vi "Test List Tests from lvlib.vi"(8 "error in (no error)":errorcluster, 11 "Test Case In":refnum<class "LUnit Test Suite Tests.lvclass">) -> (0 "error out":errorcluster, 3 "Test Case Out":refnum<class "LUnit Test Suite Tests.lvclass">)   [LabVIEW 2020, in "LUnit Test Suite Tests.lvclass"]
uses:
  LUnit Test Suite Tests.lvclass
  LUnit Test Suite Tests.lvclass/LUnit Test Suite Tests.ctl
  b74e4934-f044-4222-b3dd-fc90e6c1bd4f.vi
  source/API/Test Suite Factory/Test Suite Factory.lvclass
  source/API/LUnit Test Suite/LUnit Test Suite.lvclass
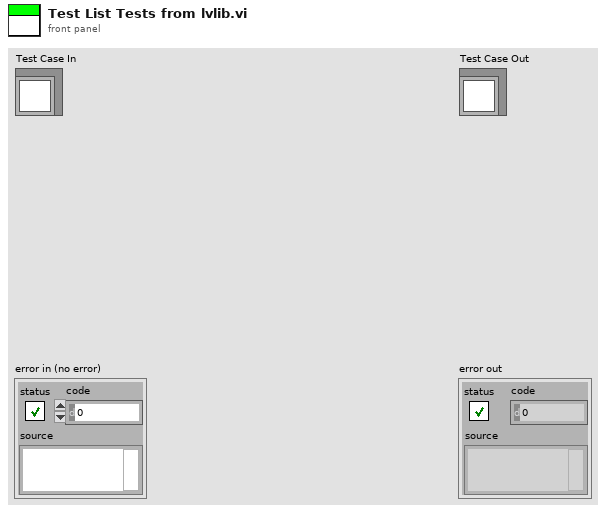
[diagram p1: front panel]
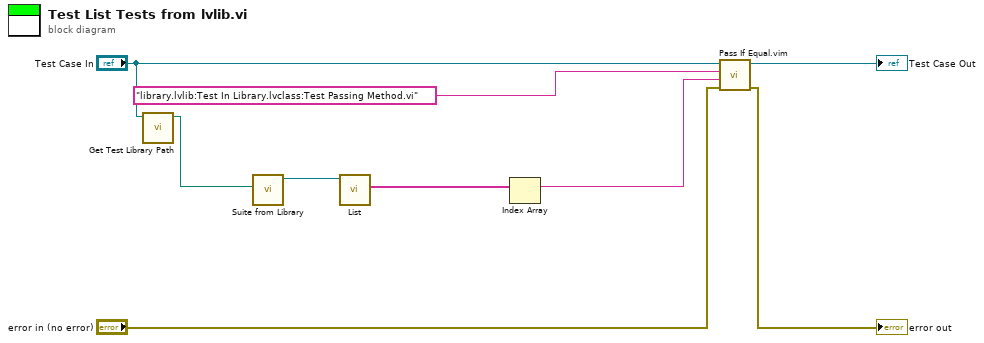
[diagram p0: block diagram]
diagram:
  n1 = call "Get Test Library Path.vi"("LUnit Test Suite Tests in"="Test Case In") -> ("lvlib path"=w1:path)  [unwired: 9 in, 1 out]
  n2 = call "Suite from Library.vi"("Library Path"=w1) -> ("LUnit Test Suite Out"=w6:refnum<class "LUnit Test Suite.lvclass">)  [unwired: 9 in, 1 out]
  n3 = call "List.vi"("LUnit Test Suite In"=w6) -> ("List of Runnables"=w5:string[])  [unwired: 9 in, 1 out]
  n4 = Index Array(array=w5) -> (element=w2:string)  [unwired: 1 in]
  n5 = call "Pass If Equal.vim"("error in (no error)"="error in (no error)", "Actual"=w2, "Expected"="library.lvlib:Test In Library.lvclass:Test Passing Method.vi" ("String"), "LUnit Test Case In"="Test Case In") -> ("error out"=→"error out":errorcluster, "LUnit Test Case Out"=→"Test Case Out":refnum<class "LUnit Test Suite Tests.lvclass">)  [unwired: 6 in]
